vi "tvac_gui_v2.vi"() -> ()   [LabVIEW 2017]
uses:
  test_indicator.ctl
  <vilib>/httpClient/ClientHandle.ctl
  msg7171_linux.llb/send single message.vi
  <vilib>/httpClient/POSTBuffer.vi
  <vilib>/httpClient/LabVIEWHTTPClient.lvlib
panel:
  out "output array":dbl[](array[numeric])
  out "deleted portion":dbl[](array[numeric])
  out "Button":u16
  in  "Tab Control":enum32{"Page 1", "Page 2"}(tab)
  in  "Zone 1":T1 {"Ring" items=["Average", "Maximum", "Minimum", ""]}
  in  "Run 2":bool
  in  "Run 3":bool
  in  "Run 4":bool
  in  "Run":bool
  out "Waveform Chart":waveform(dbl)[](graph)
  out "body":string
  out "Thermocouples":T2 {"TC 5" format="%.2g"; "TC 4" format="%.2g"; "TC 3" format="%.2g"; "TC 2" format="%.2g"; "TC 1" format="%.2g"}
  in  "exit":bool
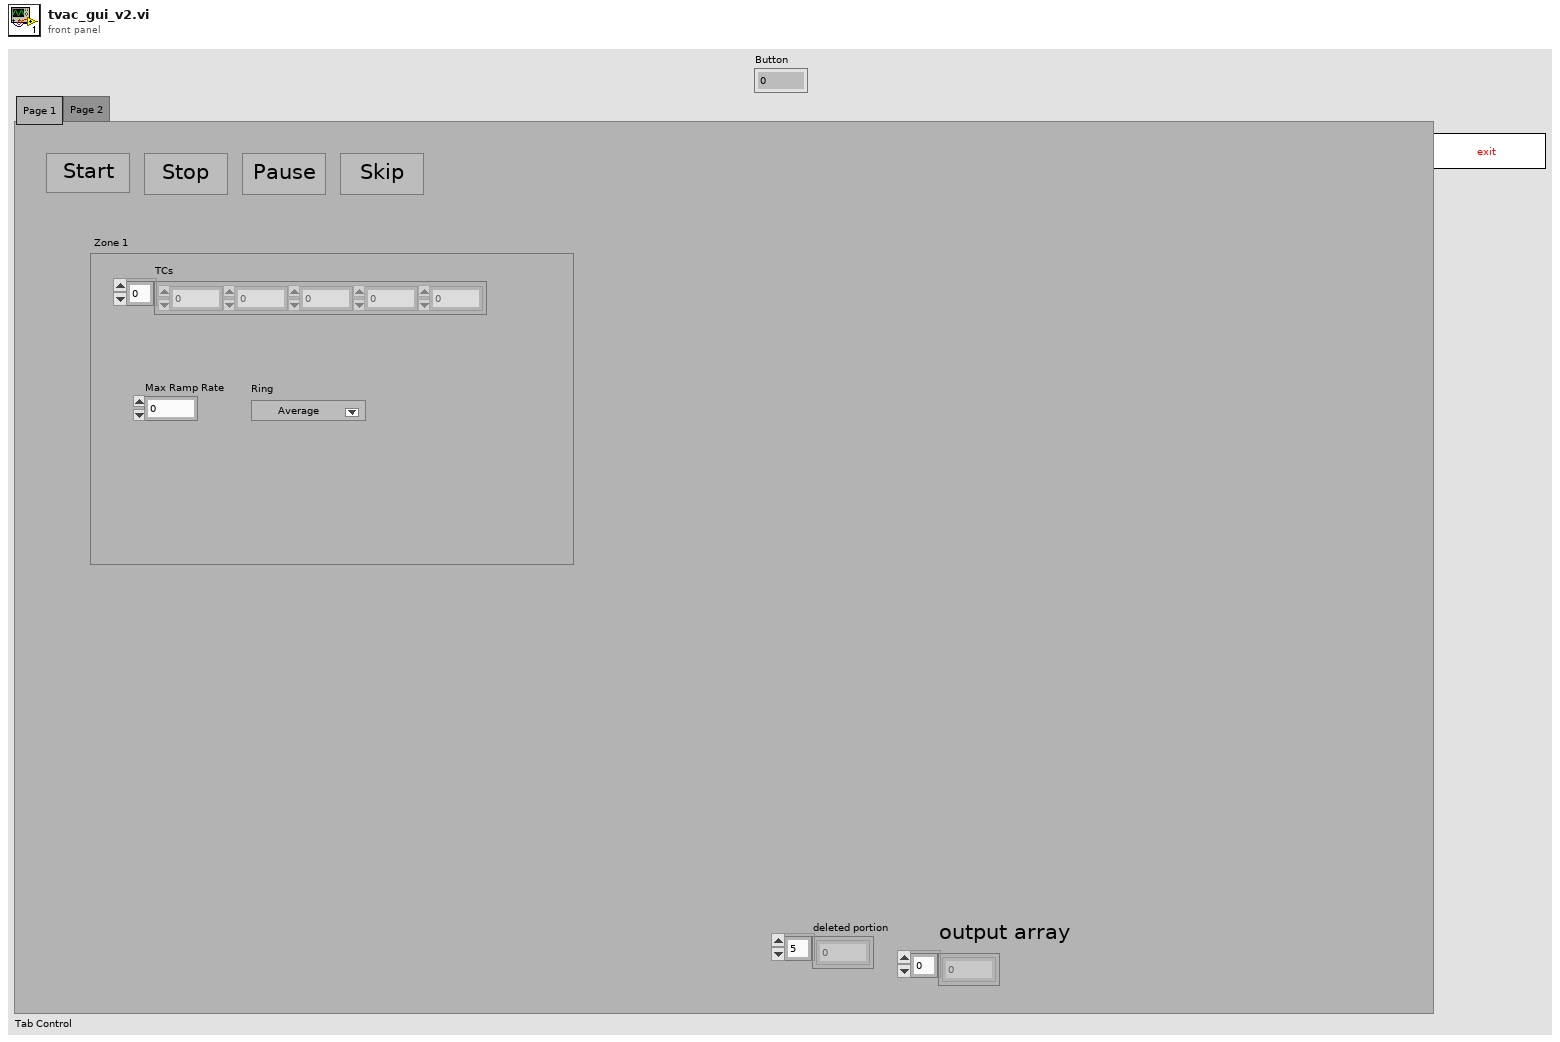
[diagram p1: front panel]
types:
  T1 = cluster{"Ring":u16, "Max Ramp Rate":dbl, "TCs":dbl[]}
  T2 = typedef "test_indicator.ctl" = cluster{"TC 1":dbl, "TC 2":dbl, "TC 3":dbl, "TC 4":dbl, "TC 5":dbl}
  T3 = typedef "LabVIEWHTTPClient.lvlib/ClientHandle.ctl" = refnum<k1>
  T4 = cluster{"go":bool, "Http session":T3, "URL prefex":string}
  T5 = typedef "LVPoint32TypeDef.ctl" = cluster{"Horizontal":i32, "Vertical":i32}
  T6 = typedef "LVPositionTypeDef.ctl" = cluster{"Left":i32, "Top":i32}
  T7 = cluster{"time":string, "tcs":cluster{"thermocouple":i32, "time":i32, "temp":i32, "working":i32}[]}
  T8 = cluster{"thermocouple":i32, "time":i32, "temp":i32, "working":i32}[]
  T9 = cluster{"thermocouple":i32, "time":i32, "temp":i32, "working":i32}
  T10 = cluster{"[0]":dbl, "[1]":dbl, "[2]":dbl, "[3]":dbl, "[4]":dbl}
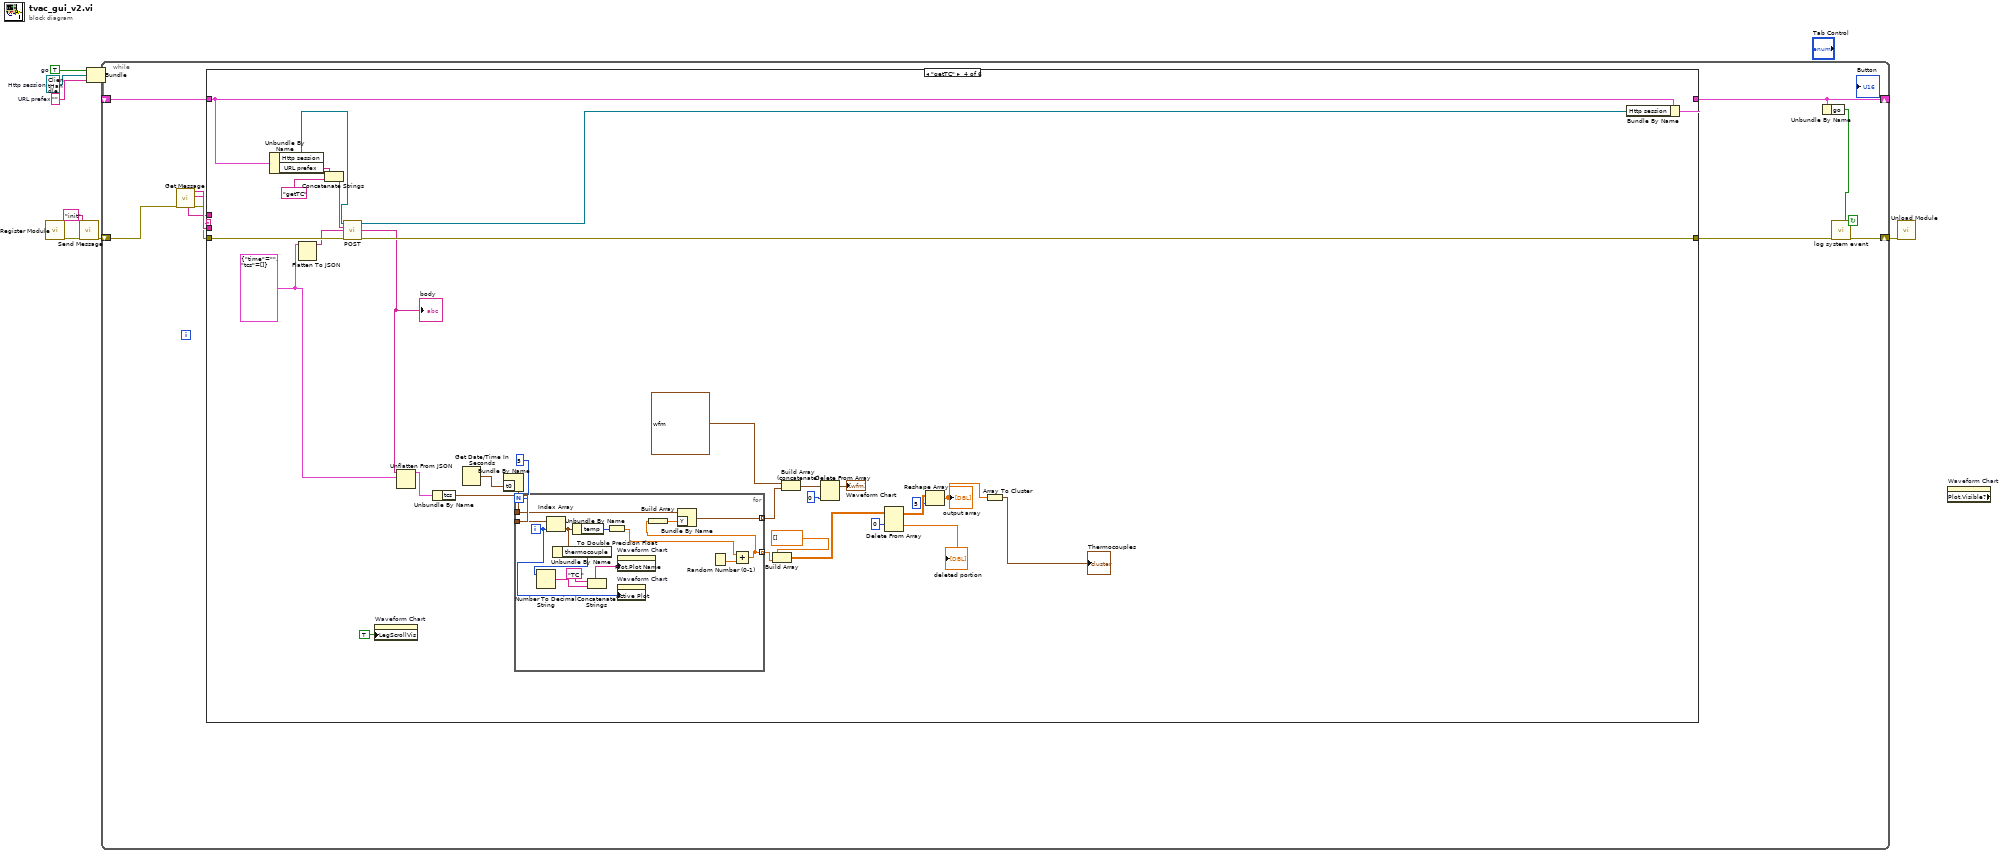
[diagram p0: block diagram]
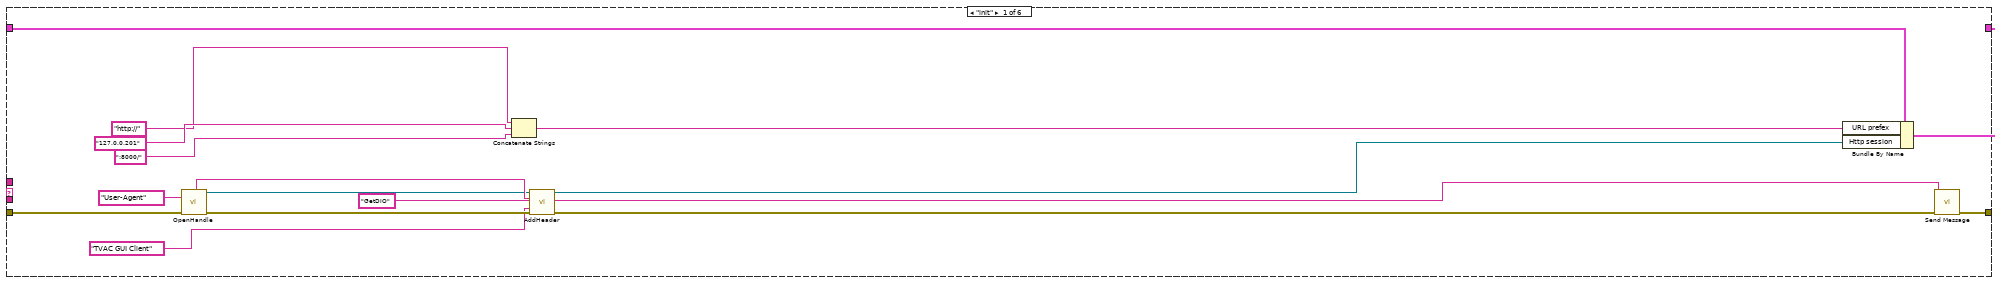
[diagram p2: hidden frame]
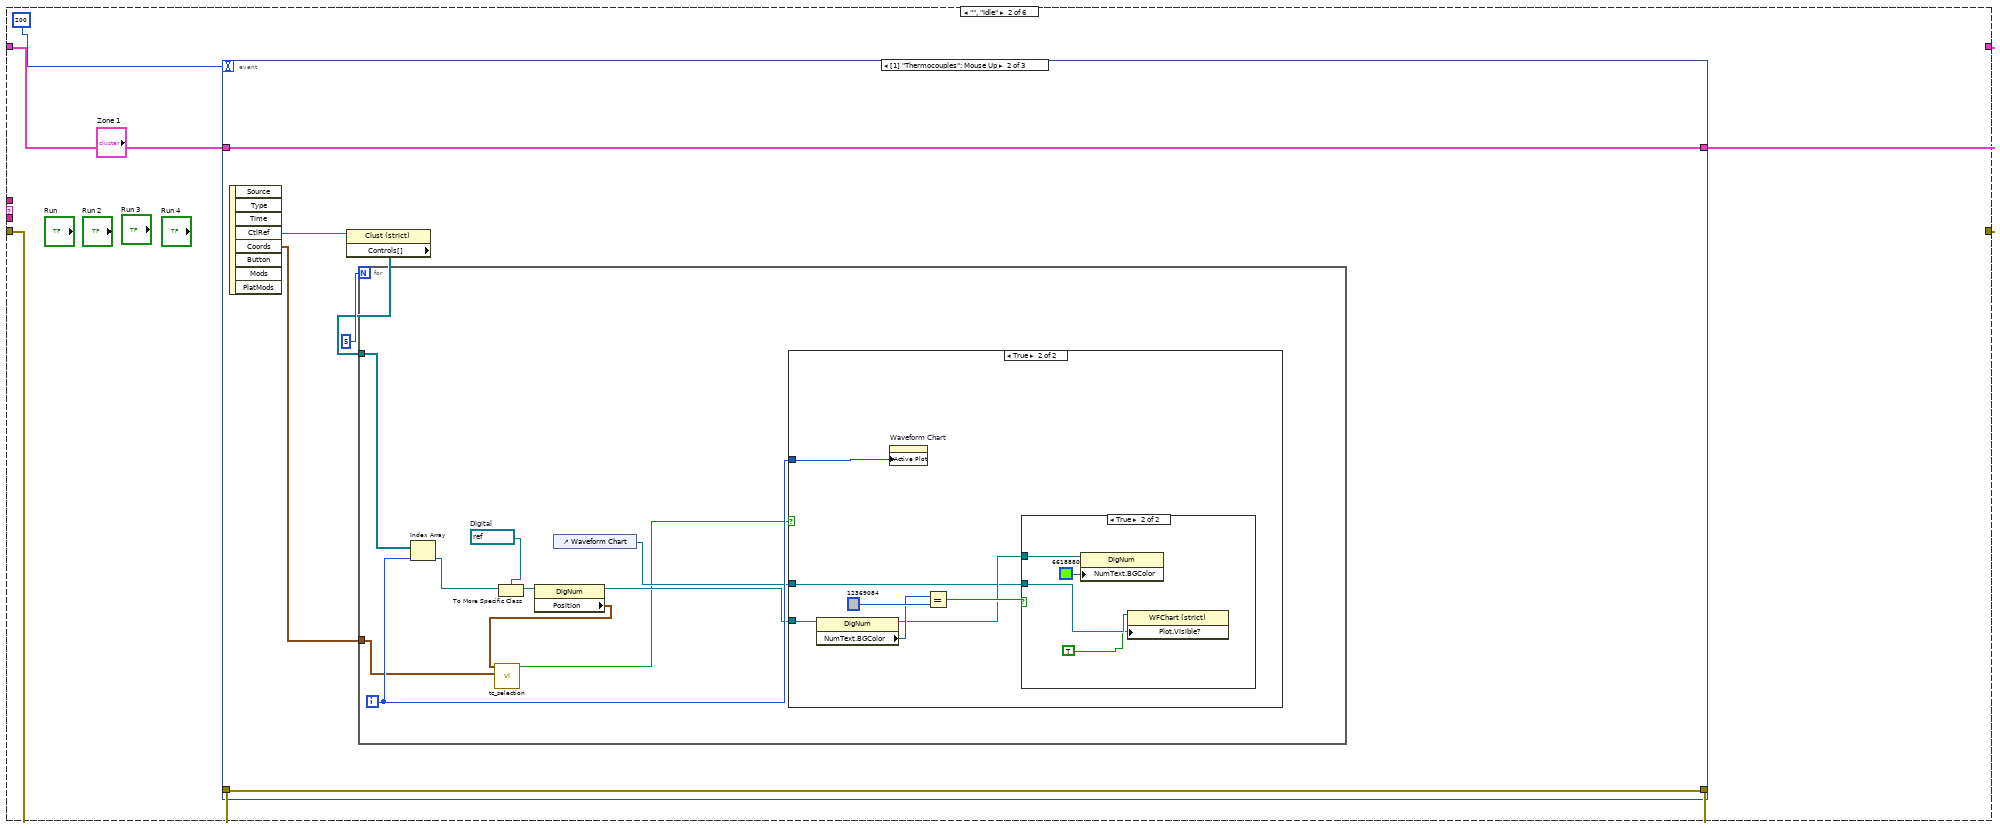
[diagram p3: hidden frame]
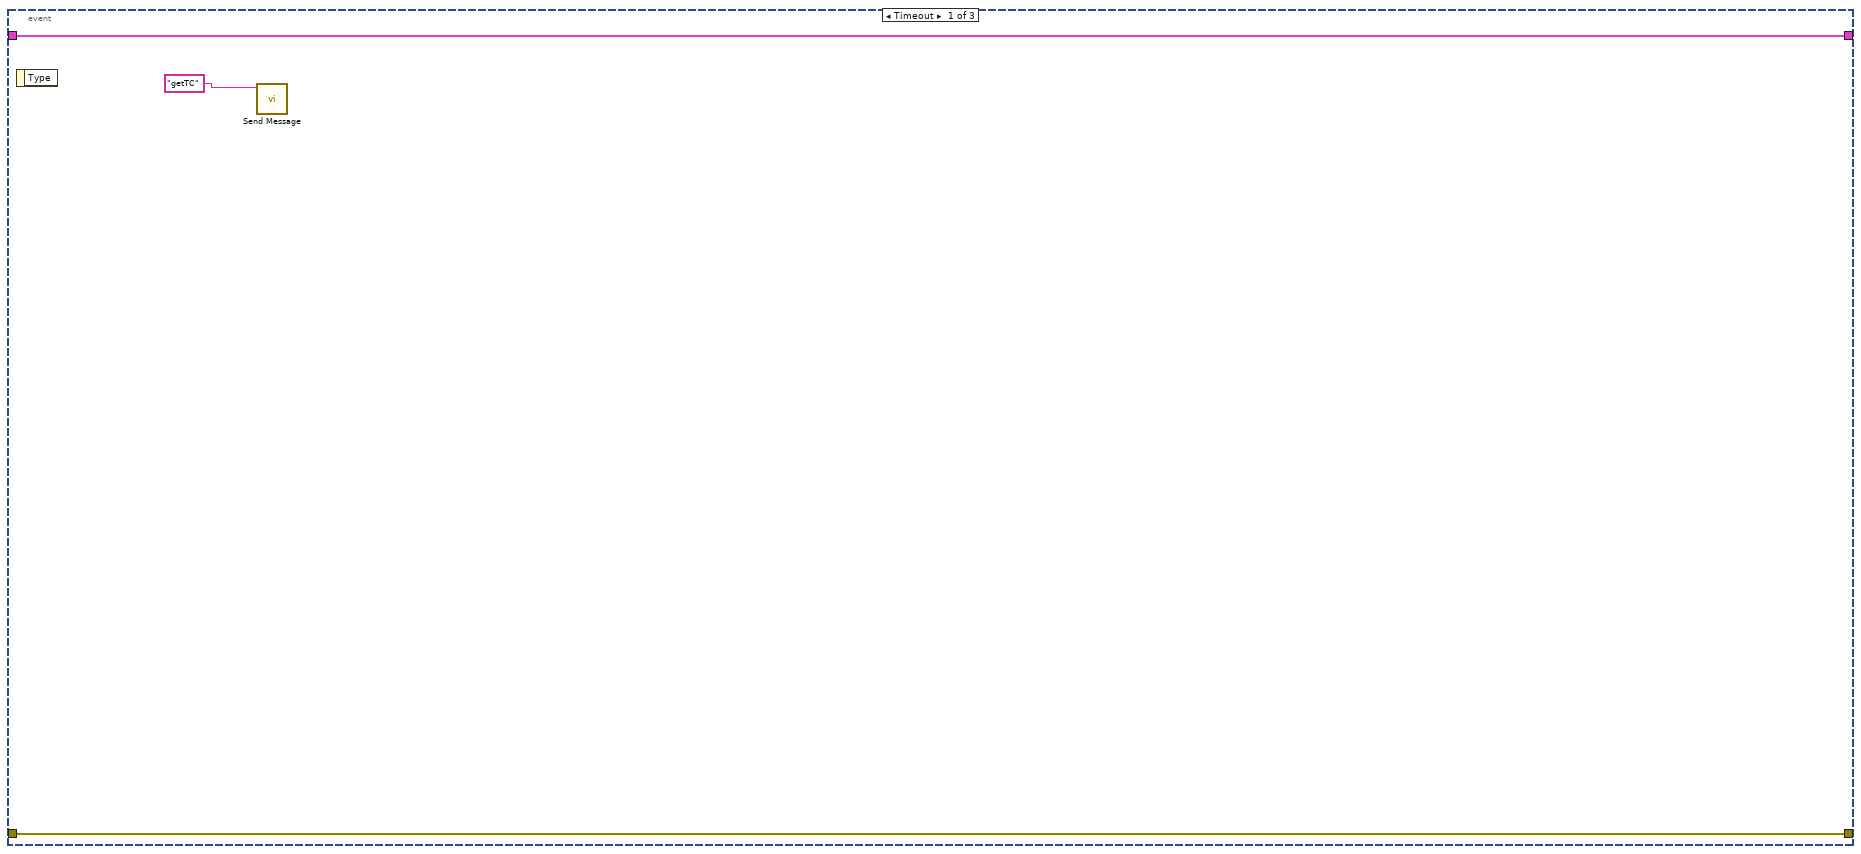
[diagram p4: hidden frame]
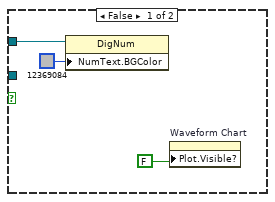
[diagram p6: hidden frame]
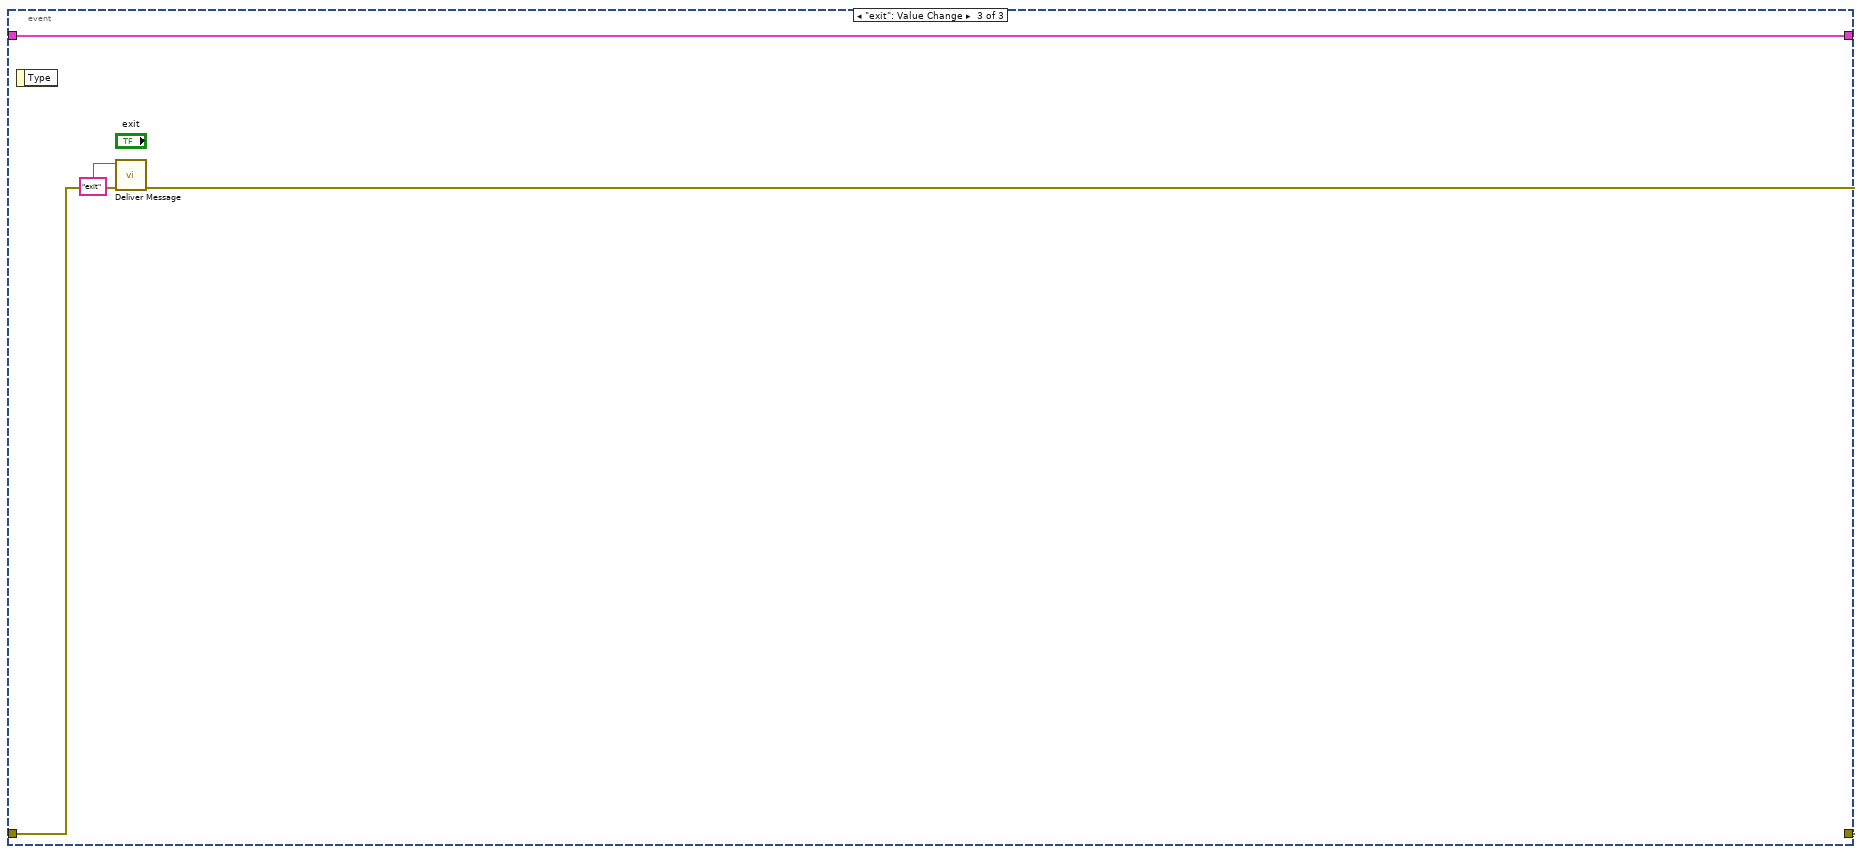
[diagram p7: hidden frame]
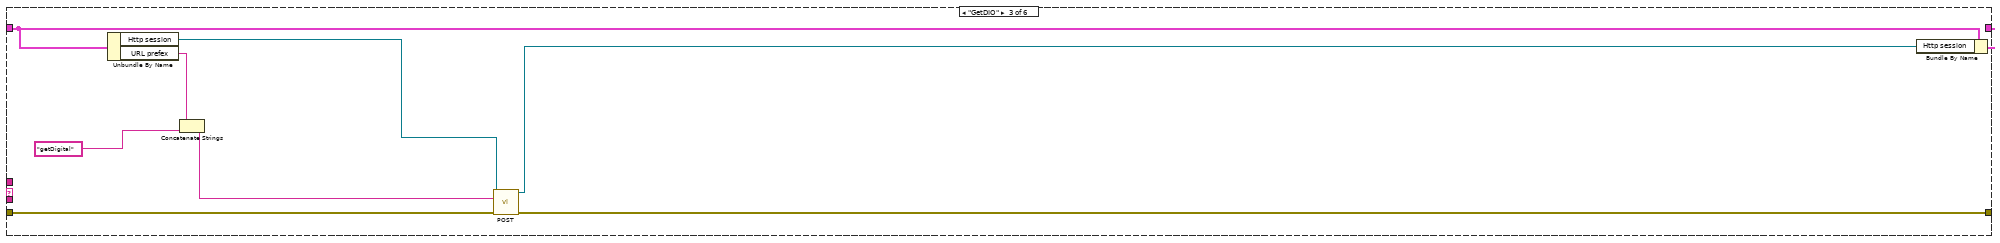
[diagram p8: hidden frame]
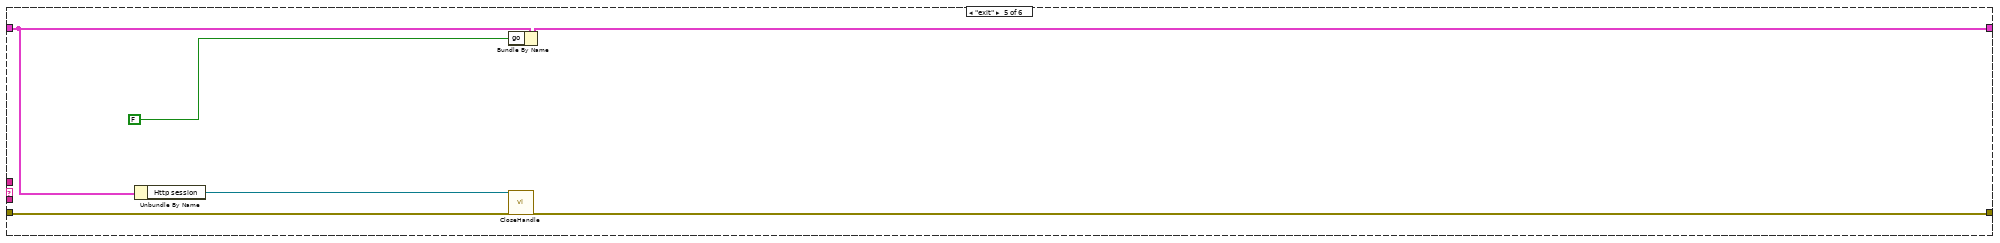
[diagram p9: hidden frame]
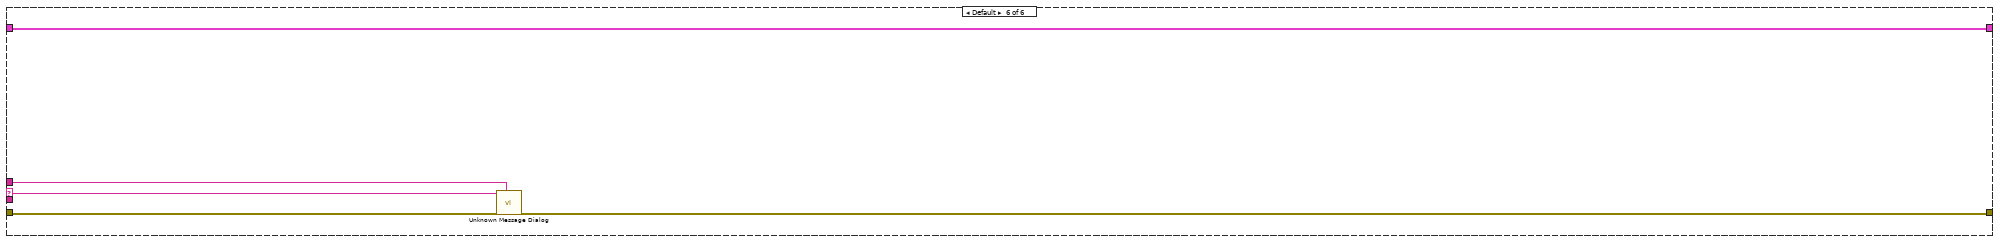
[diagram p10: hidden frame]
diagram:
  w4 = ""  # URL prefex
  w5 = T3 refnum  # Http session
  w6 = TRUE  # go
  n1 = call "Register Module.vi"() -> ("error out"=w2:errorcluster)  [unwired: 10 in, 1 out]
  n2 = call-poly "Send Message.vi"("error in (no error)"=w2, "event"="init") -> ("error out"=w1:errorcluster)  [unwired: 9 in]
  n3 = Bundle("go"=w6, "Http session"=w5, "URL prefex"=w4) -> (w8:T4)  [unwired: 1 in]
  n4 = while {
    shift-left: w8 -> [w15]
    shift-right: [w12] -> _
    shift-right: [w10] -> w7
    shift-left: w1 -> [w18]
    stop <- w11 continue-if-true
    n5 = call "Get Message.vi"("error in (no error)"=w18) -> ("error out"=w16:errorcluster, "event buffer"=w17:string, "event"=w14:string, "source"=w13:string)  [unwired: 7 in]
    n6 = case shown="\"getTC\"" w14 {
      selector: w14 -> [_ _ _ _ _ w139]
      tunnel: [w24 w35 w77 w114 w136 w141] -> w12
      tunnel: w15 -> [w33 w34 w76 w112 w131 w141]
      tunnel: w17 -> [_ _ _ _ _ _]
      tunnel: w16 -> [w28 w36 w79 w116 w134 w140]
      tunnel: w13 -> [_ _ _ _ _ w138]
      tunnel: [w20 w38 w78 w115 w133 w137] -> w9
      frame "init" {
        n7 = call <vilib>:"OpenHandle.vi"("error in (no error)"=w28) -> ("client handle out"=w29:T3, "error out"=w32:errorcluster)  [unwired: 13 in]
        n8 = Concatenate Strings("http://" ("url"), "127.0.0.201" ("Address"), ":8000/" ("url")) -> (w23:string)
        n9 = call <vilib>:"AddHeader.vi"("client handle"=w29, "header"="User-Agent", "value"="TVAC GUI Client", "error in (no error)"=w32) -> ("client handle out"=w22:T3, "error out"=w21:errorcluster)  [unwired: 10 in]
        n10 = Bundle By Name(cluster=w33, "URL prefex"=w23, "Http session"=w22) -> (w24:T4)
        n11 = call-poly "Send Message.vi"("error in (no error)"=w21, "event"="GetDIO") -> ("error out"=w20:errorcluster)  [unwired: 9 in]
      }
      frame "", "Idle" {
        n12 = event shown="[1] \"Thermocouples\": Mouse Up" {
          selector: _ -> [_ _ _]
          dyn-events: _ -> [_ _ _]
          timeout: 200 ("milliseconds to wait") -> [_ _ _]
          tunnel: w36 -> [w40 w47 w75]
          tunnel: [w40 w47 w74] -> w38
          tunnel: [w41 w46 w72] -> w35
          tunnel: w34 -> [w41 w46 w72]
          event Timeout {
            n13 = event-data() -> ()  [unwired: 1 in, 1 out]
            n14 = call-poly "Send Message.vi"("event"="getTC") -> ()  [unwired: 10 in, 1 out]
          }
          event Mouse Up {
            n15 = event-data() -> ("CtlRef"=w45:refnum<vi>, "Coords"=w42:T5)  [unwired: 1 in, 6 out]
            n16 = property class="Clust (strict)"(reference=w45) -> ("Controls[]"=w43:refnum<vi>[])  [unwired: 1 in, 2 out]
            n17 = for {
              N: 5 -> [_]
              tunnel: w43 -> [w57]
              tunnel: w42 -> [w48]
              i -> [w52]
              w55 = refnum<vi> refnum  # Digital
              n18 = Index Array(array=w57, index=w52) -> (element=w56:refnum<vi>)
              n19 = To More Specific Class(target class=w55, reference=w56) -> (specific class reference=w53:refnum<vi>)  [unwired: 1 in, 1 out]
              n20 = property class="DigNum"(reference=w53) -> (reference out=w51:refnum<vi>, "Position"=w54:T6)  [unwired: 1 in, 1 out]
              n21 = call "tc_selection.vi"("Coords"=w48, "Position"=w54) -> ("Boolean"=w49:bool)  [unwired: 9 in]
              n22 = control-ref of="Waveform Chart"() -> (w50:refnum<vi>)
              n23 = case shown="True" w49 {
                tunnel: w51 -> [_ w62]
                tunnel: w50 -> [_ w59]
                tunnel: w52 -> [_ w58]
                frame False {
                }
                frame True {
                  n24 = property class="DigNum"(reference=w62) -> (reference out=w60:refnum<vi>, "NumText.BGColor"=w61:u32)  [unwired: 1 in, 1 out]
                  n25 = property on="Waveform Chart" class="WFChart (strict)"("Active Plot"=w58) -> ()  [unwired: 2 in, 2 out]
                  n26 = Equal?(x=w61, y=u32 12369084) -> (x = y?=w63:bool)
                  n27 = case shown="True" w63 {
                    tunnel: w60 -> [w66 w70]
                    tunnel: w59 -> [_ w69]
                    frame False {
                      n28 = property class="DigNum"(reference=w66, "NumText.BGColor"=u32 12369084) -> ()  [unwired: 1 in, 2 out]
                      n29 = property on="Waveform Chart" class="WFChart (strict)"("Plot.Visible?"=FALSE ("Plot.Visible")) -> ()  [unwired: 2 in, 2 out]
                    }
                    frame True {
                      n30 = property class="DigNum"(reference=w70, "NumText.BGColor"=u32 6618880) -> ()  [unwired: 1 in, 2 out]
                      n31 = property class="WFChart (strict)"(reference=w69, "Plot.Visible?"=TRUE ("Plot.Visible")) -> ()  [unwired: 1 in, 2 out]
                    }
                  }
                }
              }
            }
          }
          event "exit": Value Change {
            n32 = event-data() -> ()  [unwired: 1 in, 1 out]
            n33 = call "Deliver Message.vi"("error in (no error)"=w75, "event"="exit") -> ("error out"=w74:errorcluster)  [unwired: 9 in]
          }
        }
      }
      frame "GetDIO" {
        n34 = Unbundle By Name(w76) -> ("Http session"=w83:T3, "URL prefex"=w81:string)
        n35 = Concatenate Strings(w81, "getDigital" ("url")) -> (w82:string)
        n36 = call-poly <vilib>:"POST.vi"("client handle"=w83, "url"=w82, "error in (no error)"=w79) -> ("client handle out"=w84:T3, "error out"=w78:errorcluster)  [unwired: 9 in, 2 out]
        n37 = Bundle By Name(cluster=w76, "Http session"=w84) -> (w77:T4)
      }
      frame "getTC" {
        w105 = T7 {"time"="", "tcs"=[]}
        n38 = Unbundle By Name(w112) -> ("Http session"=w111:T3, "URL prefex"=w109:string)
        n39 = Flatten To JSON(anything=w105) -> (JSON string=w107:string)  [unwired: 2 in, 1 out]
        n40 = Concatenate Strings(w109, "getTC" ("url")) -> (w110:string)
        n41 = call-poly <vilib>:"POST.vi"("client handle"=w111, "url"=w110, "buffer"=w107, "error in (no error)"=w116) -> ("client handle out"=w113:T3, "body"=w106:string, "error out"=w115:errorcluster)  [unwired: 8 in, 1 out]
        "body" <- w106
        n42 = property on="Waveform Chart" class="WFChart (strict)"("LegScrollVis"=TRUE ("Legend:Scrollbar Visible")) -> ()  [unwired: 2 in, 2 out]
        n43 = Unflatten From JSON(JSON string=w106, type and defaults=w105) -> (value=w104:T7)  [unwired: 5 in, 1 out]
        n44 = Unbundle By Name(w104) -> ("tcs"=w103:T8)
        n45 = Get Date/Time In Seconds() -> (seconds since 1Jan1904=w98:timestamp)
        n46 = Bundle By Name("t0"=w98) -> (w97:waveform(dbl))  [unwired: 1 in]
        n47 = for {
          N: 5 -> [_]
          tunnel: w103 -> [w130]
          tunnel: w97 -> [w128]
          tunnel: [w129] -> w96 mode=indexing
          tunnel: [w117] -> w94 mode=indexing
          i -> [w122]
          n48 = Index Array(array=w130, index=w122) -> (element=w127:T9)
          n49 = Unbundle By Name(w127) -> ("thermocouple"=w125:i32)
          n50 = Number To Decimal String(number=w125) -> (decimal integer string=w126:string)  [unwired: 1 in]
          n51 = Unbundle By Name(w127) -> ("temp"=w121:i32)
          n52 = Concatenate Strings("TC " ("string"), w126) -> (w123:string)
          n53 = To Double Precision Float(number=w121) -> (double precision float=w118:dbl)
          n54 = property on="Waveform Chart" class="WFChart (strict)"("Plot.Plot Name"=w123) -> ()  [unwired: 2 in, 2 out]
          n55 = property on="Waveform Chart" class="WFChart (strict)"("Active Plot"=w122) -> ()  [unwired: 2 in, 2 out]
          n56 = Random Number (0-1)() -> (number: 0 to 1=w119:dbl)
          n57 = Add(x=w118, y=w119) -> (x+y=w117:dbl)
          n58 = Build Array(w117) -> (w120:dbl[])
          n59 = Bundle By Name(cluster=w128, "Y"=w120) -> (w129:waveform(dbl))
        }
        n60 = Build Array(dbl[] [] ("Y"), w94) -> (w92:dbl[][])
        n61 = Build Array (concatenate)(waveform(dbl) {"t0"=timestamp(0 s since 1904-01-01), "dt"=1.0, "Y"=[]} ("element"), w96) -> (w100:waveform(dbl)[])
        n62 = Delete From Array(array=w100, index=0) -> (array with subset deleted=→"Waveform Chart":waveform(dbl)[])  [unwired: 1 in, 1 out]
        n63 = Delete From Array(array=w92, index (row)=0) -> (deleted portion=→"deleted portion":dbl[], array with subset deleted=w90:dbl[][])  [unwired: 2 in]
        n64 = Reshape Array(w90, 5 ("dimension size")) -> (w86:dbl[])
        "output array" <- w86
        n65 = Array To Cluster(array=w86) -> (cluster=→"Thermocouples":T10)
        n66 = Bundle By Name(cluster=w112, "Http session"=w113) -> (w114:T4)
      }
      frame "exit" {
        n67 = Unbundle By Name(w131) -> ("Http session"=w132:T3)
        n68 = Bundle By Name(cluster=w131, "go"=FALSE ("Bundle Element")) -> (w136:T4)
        n69 = call <vilib>:"CloseHandle.vi"("client handle"=w132, "error in (no error)"=w134) -> ("error out"=w133:errorcluster)  [unwired: 13 in]
      }
      frame Default {
        n70 = call "Unknown Message Dialog.vi"("source"=w138, "error in (no error)"=w140, "event name"=w139) -> ("error out"=w137:errorcluster)  [unwired: 8 in]
      }
    }
    n71 = Unbundle By Name(w12) -> ("go"=w11:bool)
    n72 = call "log system event.vi"("error in (no error)"=w9) -> ("error out"=w10:errorcluster)  [unwired: 9 in, 1 out]
  }
  n73 = call "Unload Module.vi"("error in (no error)"=w7) -> ()  [unwired: 10 in, 1 out]
  n74 = property on="Waveform Chart" class="WFChart (strict)" props=["Plot", "Visible?"]() -> ()  [unwired: 2 in, 3 out]
